vi "selector_compose_cmd.vi"(5 "Repeated Capability":string, 6 "Selector Name":string, 7 "Attribute":T1={"Identifier"="", "Descriptive name"="", "Data Type"=enum."Integer 32", "Command"="", "Access"=2, "Range Table"="", "Read Callback"="", "Write Callback"="", "Range Callback"="", "Check Callback"="", "Rngtable Callback"="", "Coerce Callback"="", "Supported Models"="", "Instrument Options"="", "Repeated Capabilities"="", "Check Status Callback"="", "Index"=0, "Flag: OPC Wait"=FALSE, "Flag: Dont check status"=FALSE, "Flag: Cache Only"=FALSE} {"Access" items=["Read Only", "Write Only", "Read/Write"]}, 8 "error in":errorcluster, 10 "Selector Attribute ID":string, 11 "VISA resource name":refnum<visa-resource-name>) -> (0 "error out":errorcluster, 2 "Attribute out":T1={"Identifier"="", "Descriptive name"="", "Data Type"=enum."Integer 32", "Command"="", "Access"=2, "Range Table"="", "Read Callback"="", "Write Callback"="", "Range Callback"="", "Check Callback"="", "Rngtable Callback"="", "Coerce Callback"="", "Supported Models"="", "Instrument Options"="", "Repeated Capabilities"="", "Check Status Callback"="", "Index"=0, "Flag: OPC Wait"=FALSE, "Flag: Dont check status"=FALSE, "Flag: Cache Only"=FALSE} {"Access" items=["Read Only", "Write Only", "Read/Write"]}, 3 "VISA resource name out":refnum<visa-resource-name>)   [LabVIEW 2014, in "rszvl_rsidr_core.lvlib"]
uses:
  rszvl_rsidr_core.lvlib
  type_Attribute.ctl
  type_Attribute_Data_Type.ctl
  type_Error_Codes.ctl
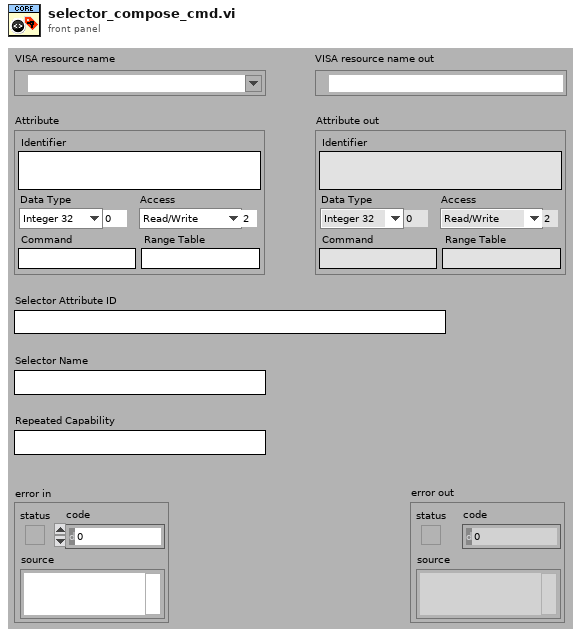
[diagram p1: front panel]
types:
  T1 = typedef "rszvl_rsidr_core.lvlib/type_Attribute.ctl" = cluster{"Identifier":string, "Descriptive name":string, "Data Type":T2, "Command":string, "Access":u16, "Range Table":string, "Read Callback":string, "Write Callback":string, "Range Callback":string, "Check Callback":string, "Rngtable Callback":string, "Coerce Callback":string, "Supported Models":string, "Instrument Options":string, "Repeated Capabilities":string, "Check Status Callback":string, "Index":i32, "Flag: OPC Wait":bool, "Flag: Dont check status":bool, "Flag: Cache Only":bool}
  T2 = typedef "rszvl_rsidr_core.lvlib/type_Attribute_Data_Type.ctl" = enum16{"Integer 32", "Double", "String", "Boolean", "None", "Integer 64"}
  T3 = typedef "rszvl_rsidr_core.lvlib/type_Error_Codes.ctl" = enum16{"No_error", "VISA_err_ResourceNotFound", "VISA_err_Timeout", "VISA_warn_MoreDataAvailable", "RS_err_MissingCallback", "RS_err_InvalidAttribute", "RS_err_InvalidValue", "RS_err_UnknownResource", "RS_err_AlreadyInitialized", "RS_err_InstrumentStatus", "RS_err_BadRepCapName", "RS_err_TypesMismatch", "RS_err_ValueNotSupported", "RS_err_InvalidRngTable", "RS_err_IDqueryFail", "RS_err_UnexpResponse", "VISA_warn_ConfigNotLoaded", "RS_err_AttributeNotReadable", "RS_err_AttributeNotWritable", "RS_err_InstrumentType", "RS_err_InstrumentOption", "VISA_err_InvalidSize", "RS_err_ReliabilityIndicator", "VISA_warn_UnknownStatus", "VISA_warn_TermCharRead", "VISA_err_IO_error"}
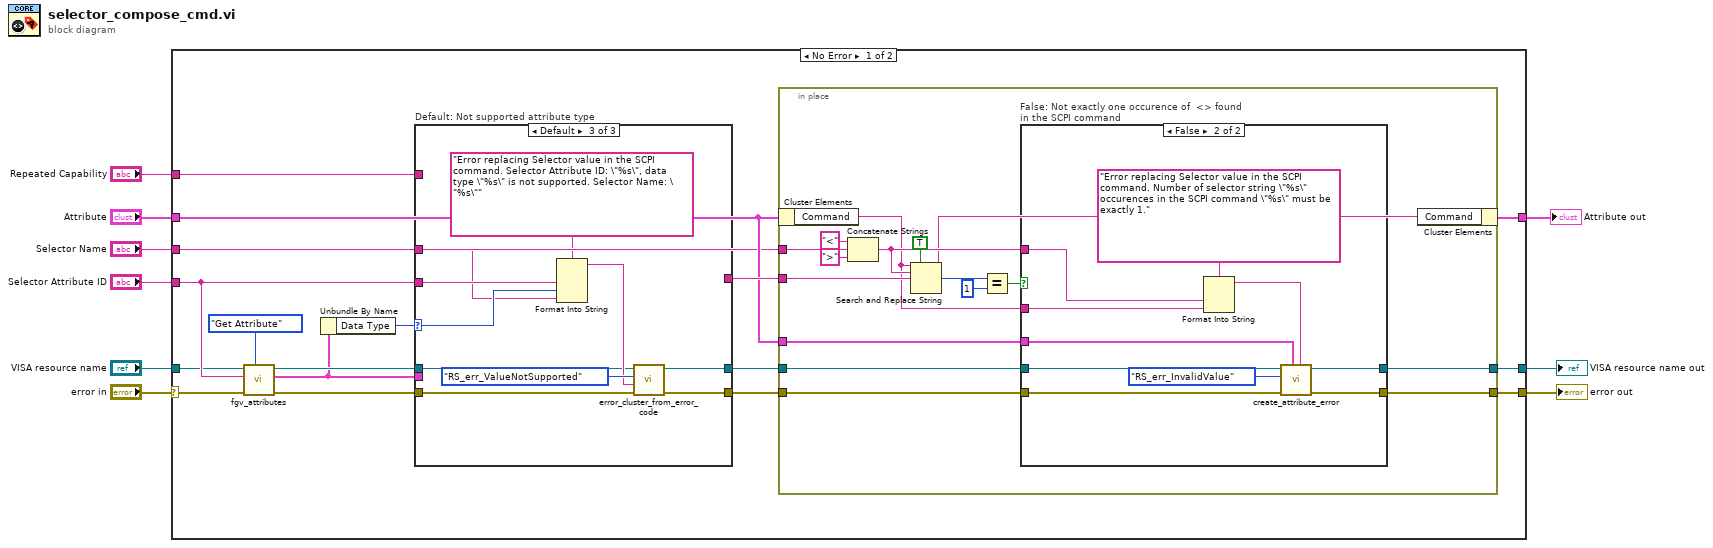
[diagram p0: block diagram]
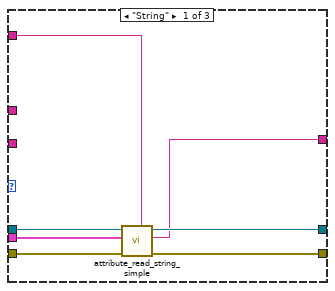
[diagram p3: hidden frame]
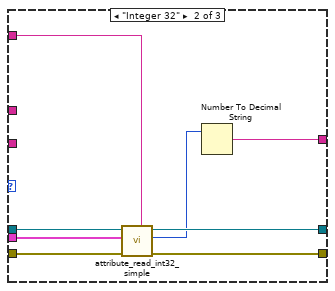
[diagram p4: hidden frame]
diagram:
  n1 = case shown="No Error" "error in" {
    selector: "error in" -> [w22 w81]
    tunnel: [w12 w79] -> w1
    tunnel: [w14 w81] -> w3
    tunnel: "VISA resource name" -> [w20 w80]
    tunnel: [w13 w80] -> w9
    tunnel: "Selector Attribute ID" -> [w23 _]
    tunnel: "Selector Name" -> [w10 _]
    tunnel: "Repeated Capability" -> [w18 _]
    tunnel: "Attribute" -> [w11 w79]
    frame No Error {
      n2 = call "fgv_attributes.vi"("Operation"=enum16{"Initialize", "Get Attribute"}."Get Attribute", "error in"=w22, "Attribute ID in"=w23) -> ("error out"=w21:errorcluster, "Attribute out"=w19:T1)  [unwired: 6 in, 1 out]
      n3 = Unbundle By Name(w19) -> ("Data Type"=w24:T2)
      n4 = case "Default: Not supported attribute type" shown="Default" w24 {
        selector: w24 -> [_ _ w70]
        tunnel: w21 -> [w60 w68 w73]
        tunnel: [w58 w66 w77] -> w15
        tunnel: w23 -> [_ _ w75]
        tunnel: w20 -> [w59 w67 w72]
        tunnel: w19 -> [w57 w65 _]
        tunnel: w18 -> [w56 w64 _]
        tunnel: [w55 w63 w71] -> w16
        tunnel: [w54 w61 _] -> w17
        tunnel: w10 -> [_ _ w69]
        frame "String" {
          n5 = call "attribute_read_string_simple.vi"("Repeated Capability"=w56, "Attribute"=w57, "error in"=w60, "VISA resource name"=w59) -> ("error out"=w58:errorcluster, "string out"=w54:string, "VISA resource name out"=w55:refnum<visa-resource-name>)  [unwired: 5 in]
        }
        frame "Integer 32" {
          n6 = call "attribute_read_int32_simple.vi"("Repeated Capability"=w64, "Attribute"=w65, "error in"=w68, "VISA resource name"=w67) -> ("error out"=w66:errorcluster, "int32 out"=w62:i32, "VISA resource name out"=w63:refnum<visa-resource-name>)  [unwired: 5 in]
          n7 = Number To Decimal String(number=w62) -> (decimal integer string=w61:string)  [unwired: 1 in]
        }
        frame Default {
          n8 = Format Into String(format string="Error replacing Selector value in the SCPI command. Selector Attribute ID: \"%s\", data type \"%s\" is not supported. Selector Name: \"%s\"", w75, w70, w69) -> (resulting string=w74:string)  [unwired: 2 in, 1 out]
          n9 = call "error_cluster_from_error_code.vi"("error in"=w73, "error message (\"\")"=w74, "Error Enum in"=type_Error_Codes."RS_err_ValueNotSupported", "VISA resource name"=w72) -> ("error out"=w77:errorcluster, "VISA resource name out"=w71:refnum<visa-resource-name>)  [unwired: 6 in]
        }
      }
      n10 = in-place "In Place Element Structure" {
        in-place-border: w10 -> [w40]
        in-place-border: w17 -> [w37]
        in-place-border: w16 -> [w32]
        in-place-border: w15 -> [w31]
        in-place-border: [w30] -> w14
        in-place-border: [w29] -> w13
        in-place-border: w11 -> [w26]
        n11 = in-place-cluster #1 ("Unbundle / Bundle Elements")(w11) -> ("Command"=w28:string)
        n12 = Concatenate Strings("<", w40, ">") -> (w33:string)
        n13 = Search and Replace String(replace all?=TRUE ("replace all? (F)"), input string=w28, search string=w33, replace string=w37) -> (result string=w27:string, number of replacements=w36:i32)  [unwired: 4 in, 2 out]
        n14 = Equal?(x=w36, y=1) -> (x = y?=w34:bool)
        n15 = case "False: Not exactly one occurence of  <> found in the SCPI command" shown="False" w34 {
          tunnel: w31 -> [w42 w50]
          tunnel: [w42 w52] -> w30
          tunnel: w32 -> [w43 w49]
          tunnel: [w43 w48] -> w29
          tunnel: w33 -> [_ w47]
          tunnel: w28 -> [_ w46]
          tunnel: w26 -> [_ w45]
          frame True {
          }
          frame False {
            n16 = Format Into String(format string="Error replacing Selector value in the SCPI command. Number of selector string \"%s\" occurences in the SCPI command \"%s\" must be exactly 1.", w47, w46) -> (resulting string=w44:string)  [unwired: 2 in, 1 out]
            n17 = call "create_attribute_error.vi"("Error Elaboration (\"\")"=w44, "Attribute"=w45, "error in"=w50, "Error Enum in"=type_Error_Codes."RS_err_InvalidValue", "VISA resource name"=w49) -> ("error out"=w52:errorcluster, "VISA resource name out"=w48:refnum<visa-resource-name>)  [unwired: 5 in]
          }
        }
        n18 = in-place-cluster #1 ("Unbundle / Bundle Elements")("Command"=w27) -> (w12:T1)
      }
    }
    frame Error {
    }
  }
  "error out" <- w3
  "VISA resource name out" <- w9
  "Attribute out" <- w1
